vi "JSON String for Simulink Models.vi"() -> ()   [LabVIEW 2018]
uses:
  NistPluggableModules/AcPwr/AcPwrPlugins/ChromaAcLoadClass/TypeDefs/Measurements.ctl
  NistPluggableModules/AcPwr/AcPwrPlugins/ChromaAcLoadClass/TypeDefs/MeasurementType.ctl
  NistPluggableModules/AcPwr/AcPwrShared/clMeasurmentData.ctl
  <vilib>/addons/_JKI.lib/Serialization/JSON/JKI JSON Serialization.lvlib
  NistPluggableModules/AcPwr/AcPwrPlugins/ChromaAcLoadClass/ChromaAcLoad.lvclass
  NistPluggableModules/AcPwr/AcPwrShared/AcPwrShared.lvlib
panel:
  in  "MeasurmentDataCluster":T1={"MeasName"="", "XML Data"="", "WaveformData"=[{"t0"=timestamp(0 s since 1904-01-01), "dt"=1.0, "Y"=[5.0]}, {"t0"=timestamp(0 s since 1904-01-01), "dt"=1.0, "Y"=[10.0]}]}
  in  "Measurements":T2=[{"Handle"="CHROMA0", "Name"="", "Enabled"=TRUE, "Measurement Value"=0.0, "Hold Peak Current Measurement"=FALSE, "btnMeasFetch"=TRUE, "ProtectionStatusString"="", "Measurement Type"=enum."Voltage (Vrms or V)"}, {"Handle"="CHROMA0", "Name"="", "Enabled"=TRUE, "Measurement Value"=0.0, "Hold Peak Current Measurement"=FALSE, "btnMeasFetch"=TRUE, "ProtectionStatusString"="", "Measurement Type"=enum."Current (Arms or A)"}]
  out "JSON String 2":string="{\r\n    \"MeasName\":\"\",\r\n    \"XML Data\":\"\",\r\n    \"WaveformData\":[\r\n                {\r\n            \"t0\":\"1904-01-01T00:00:00.000Z\",\r\n            \"dt\":1.00000000000000,\r\n            \"y\":[\r\n                5.00000000000000\r\n            ]\r\n        },\r\n                {\r\n            \"t0\":\"1904-01-01T00:00:00.000Z\",\r\n            \"dt\":1.00000000000000,\r\n            \"y\":[\r\n                10.0000000000000\r\n            ]\r\n        }\r\n    ]\r\n}"
  out "xml string":string="<Cluster>\r\n<Name>Device(s)Settings</Name>\r\n<NumElts>6</NumElts>\r\n<EW>\r\n<Name>Configuration Mode</Name>\r\n<Choice>Constant Voltage (DC)</Choice>\r\n<Choice>Constant Power (DC)</Choice>\r\n<Choice>Constant Power (AC)</Choice>\r\n<Choice>Constant Current (DC)</Choice>\r\n<Choice>Constant Current (AC)</Choice>\r\n<Choice>Constant Resistance (DC)</Choice>\r\n<Choice>Constant Resistance (AC)</Choice>\r\n<Choice>Rectified Mode (DC)</Choice>\r\n<Choice>Inrush (AC)</Choice>\r\n<Choice>RLC CP (AC)</Choice>\r\n<Choice>RLC (AC)</Choice>\r\n<Val>1</Val>\r\n</EW>\r\n<Array>\r\n<Name>Phases</Name>\r\n<Dimsize>1</Dimsize>\r\n<Cluster>\r\n<Name>Config</Name>\r\n<NumElts>23</NumElts>\r\n<String>\r\n<Name>Handle</Name>\r\n<Val>CHROMA0</Val>\r\n</String>\r\n<String>\r\n<Name>Name</Name>\r\n<Val></Val>\r\n</String>\r\n<I32>\r\n<Name>Phase Select</Name>\r\n<Val>0</Val>\r\n</I32>\r\n<String>\r\n<Name>Instrument Options</Name>\r\n<Val>Simulate=0,RangeCheck=1,QueryInstrStatus=1,Cache=0</Val>\r\n</String>\r\n<Boolean>\r\n<Name>id query (T)</Name>\r\n<Val>1</Val>\r\n</Boolean>\r\n<Boolean>\r\n<Name>reset device (T)</Name>\r\n<Val>1</Val>\r\n</Boolean>\r\n<Boolean>\r\n<Name>Load Short Circuited</Name>\r\n<Val>0</Val>\r\n</Boolean>\r\n<Boolean>\r\n<Name>Line Synchronization</Name>\r\n<Val>0</Val>\r\n</Boolean>\r\n<DBL>\r\n<Name>Load Current (A/Arms)</Name>\r\n<Val>1.00000000000000</Val>\r\n</DBL>\r\n<DBL>\r\n<Name>Load Voltage (V/Vrms)</Name>\r\n<Val>38.00000000000000</Val>\r\n</DBL>\r\n<DBL>\r\n<Name>Load Power (W)</Name>\r\n<Val>5.00000000000000</Val>\r\n</DBL>\r\n<DBL>\r\n<Name>Load Resistance (Ohms)</Name>\r\n<Val>1.50000000000000</Val>\r\n</DBL>\r\n<DBL>\r\n<Name>Load Current Peak Limit (A)</Name>\r\n<Val>45.00000000000000</Val>\r\n</DBL>\r\n<DBL>\r\n<Name>Load Current Limit (A/Arms)</Name>\r\n<Val>10.00000000000000</Val>\r\n</DBL>\r\n<DBL>\r\n<Name>Load Power Limit (W)</Name>\r\n<Val>1250.00000000000000</Val>\r\n</DBL>\r\n<DBL>\r\n<Name>Synch Frequency (Hz)</Name>\r\n<Val>0.00000000000000</Val>\r\n</DBL>\r\n<EW>\r\n<Name>Priority</Name>\r\n<Choice>CF Only</Choice>\r\n<Choice>PF Only</Choice>\r\n<Choice>Both (CF)</Choice>\r\n<Choice>Both (PF)</Choice>\r\n<Val>0</Val>\r\n</EW>\r\n<DBL>\r\n<Name>Crest Factor</Name>\r\n<Val>1.41400000000000</Val>\r\n</DBL>\r\n<DBL>\r\n<Name>Power Factor</Name>\r\n<Val>1.00000000000000</Val>\r\n</DBL>\r\n<Cluster>\r\n<Name>Slew Rate</Name>\r\n<NumElts>2</NumElts>\r\n<I32>\r\n<Name>Rise Slew Rate (A/ms)</Name>\r\n<Val>600</Val>\r\n</I32>\r\n<I32>\r\n<Name>Fall Slew Rate (A/ms)</Name>\r\n<Val>600</Val>\r\n</I32>\r\n</Cluster>\r\n<Cluster>\r\n<Name>LC/RLC Mode</Name>\r\n<NumElts>4</NumElts>\r\n<I32>\r\n<Name>Capacitance (uF)</Name>\r\n<Val>0</Val>\r\n</I32>\r\n<I32>\r\n<Name>Inductance (uH)</Name>\r\n<Val>0</Val>\r\n</I32>\r\n<DBL>\r\n<Name>Series Resistance (Ohm)</Name>\r\n<Val>0.00000000000000</Val>\r\n</DBL>\r\n<DBL>\r\n<Name>Parallel Resistance (Ohm)</Name>\r\n<Val>0.00000000000000</Val>\r\n</DBL>\r\n</Cluster>\r\n<Cluster>\r\n<Name>Timing</Name>\r\n<NumElts>5</NumElts>\r\n<EW>\r\n<Name>TimingOn</Name>\r\n<Choice></Choice>\r\n<Val>0</Val>\r\n</EW>\r\n<U32>\r\n<Name>Hours</Name>\r\n<Val>0</Val>\r\n</U32>\r\n<U32>\r\n<Name>Minutes</Name>\r\n<Val>0</Val>\r\n</U32>\r\n<DBL>\r\n<Name>Seconds</Name>\r\n<Val>0.00000000000000</Val>\r\n</DBL>\r\n<DBL>\r\n<Name>CutoffVoltage</Name>\r\n<Val>0.00000000000000</Val>\r\n</DBL>\r\n</Cluster>\r\n<Boolean>\r\n<Name>Connected</Name>\r\n<Val>0</Val>\r\n</Boolean>\r\n</Cluster>\r\n</Array>\r\n<String>\r\n<Name>MeasName</Name>\r\n<Val>AcPwr.ChromaAcLoad.63804-CH0</Val>\r\n</String>\r\n<String>\r\n<Name>Data Source</Name>\r\n<Val>ICDAS_Simulink_DB</Val>\r\n</String>\r\n<String>\r\n<Name>ICDAS to Model Table Name</Name>\r\n<Val>ICDAS_Simulink_DB</Val>\r\n</String>\r\n<String>\r\n<Name>Model to ICDAS Table Name</Name>\r\n<Val>ICDAS_Simulink_DB</Val>\r\n</String>\r\n</Cluster>\r\n"
  out "JSON String":string="{\r\n    \"Device(s)Settings\":{\r\n        \"Configuration Mode\":1,\r\n        \"Phases\":[\r\n            {\r\n                \"Handle\":\"CHROMA0\",\r\n                \"Name\":\"\",\r\n                \"Phase Select\":0,\r\n                \"Instrument Options\":\"Simulate=0,RangeCheck=1,QueryInstrStatus=1,Cache=0\",\r\n                \"id query (T)\":true,\r\n                \"reset device (T)\":true,\r\n                \"Load Short Circuited\":false,\r\n                \"Line Synchronization\":false,\r\n                \"Load Current (A/Arms)\":1.00000000000000,\r\n                \"Load Voltage (V/Vrms)\":38.0000000000000,\r\n                \"Load Power (W)\":5.00000000000000,\r\n                \"Load Resistance (Ohms)\":1.50000000000000,\r\n                \"Load Current Peak Limit (A)\":45.0000000000000,\r\n                \"Load Current Limit (A/Arms)\":10.0000000000000,\r\n                \"Load Power Limit (W)\":1250.00000000000,\r\n                \"Synch Frequency (Hz)\":0.00000000000000,\r\n                \"Priority\":0,\r\n                \"Crest Factor\":1.41400000000000,\r\n                \"Power Factor\":1.00000000000000,\r\n                \"Slew Rate\":{\r\n                    \"Rise Slew Rate (A/ms)\":600,\r\n                    \"Fall Slew Rate (A/ms)\":600\r\n                },\r\n                \"LC/RLC Mode\":{\r\n                    \"Capacitance (uF)\":0,\r\n                    \"Inductance (uH)\":0,\r\n                    \"Series Resistance (Ohm)\":0.00000000000000,\r\n                    \"Parallel Resistance (Ohm)\":0.00000000000000\r\n                },\r\n                \"Timing\":{\r\n                    \"TimingOn\":0,\r\n                    \"Hours\":0,\r\n                    \"Minutes\":0,\r\n                    \"Seconds\":0.00000000000000,\r\n                    \"CutoffVoltage\":0.00000000000000\r\n                },\r\n                \"Connected\":false\r\n            }\r\n        ],\r\n        \"MeasName\":\"AcPwr.ChromaAcLoad.63804-CH0\",\r\n        \"Data Source\":\"ICDAS_Simulink_DB\",\r\n        \"ICDAS to Model Table Name\":\"ICDAS_Simulink_DB\",\r\n        \"Model to ICDAS Table Name\":\"ICDAS_Simulink_DB\"\r\n    },\r\n    \"Measurements\":[\r\n        {\r\n            \"Handle\":\"CHROMA0\",\r\n            \"Name\":\"\",\r\n            \"Enabled\":true,\r\n            \"Measurement Value\":0.00000000000000,\r\n            \"Hold Peak Current Measurement\":false,\r\n            \"btnMeasFetch\":true,\r\n            \"ProtectionStatusString\":\"\",\r\n            \"Measurement Type\":0\r\n        },\r\n        {\r\n            \"Handle\":\"CHROMA0\",\r\n            \"Name\":\"\",\r\n            \"Enabled\":true,\r\n            \"Measurement Value\":0.00000000000000,\r\n            \"Hold Peak Current Measurement\":false,\r\n            \"btnMeasFetch\":true,\r\n            \"ProtectionStatusString\":\"\",\r\n            \"Measurement Type\":1\r\n        }\r\n    ]\r\n}"
  in  "Device(s)Settings":T4={"Configuration Mode"=enum."Constant Power (DC)", "Phases"=[{"Handle"="CHROMA0", "Name"="", "Phase Select"=0, "Instrument Options"="Simulate=0,RangeCheck=1,QueryInstrStatus=1,Cache=0", "id query (T)"=TRUE, "reset device (T)"=TRUE, "Load Short Circuited"=FALSE, "Line Synchronization"=FALSE, "Load Current (A/Arms)"=1.0, "Load Voltage (V/Vrms)"=38.0, "Load Power (W)"=5.0, "Load Resistance (Ohms)"=1.5, "Load Current Peak Limit (A)"=45.0, "Load Current Limit (A/Arms)"=10.0, "Load Power Limit (W)"=1250.0, "Synch Frequency (Hz)"=0.0, "Priority"=enum."CF Only", "Crest Factor"=1.414, "Power Factor"=1.0, "Slew Rate"={"Rise Slew Rate (A/ms)"=600, "Fall Slew Rate (A/ms)"=600}, "LC/RLC Mode"={"Capacitance (uF)"=0, "Inductance (uH)"=0, "Series Resistance (Ohm)"=0.0, "Parallel Resistance (Ohm)"=0.0}, "Timing"={"TimingOn"=enum."", "Hours"=0, "Minutes"=0, "Seconds"=0.0, "CutoffVoltage"=0.0}, "Connected"=FALSE}], "MeasName"="AcPwr.ChromaAcLoad.63804-CH0", "Data Source"="ICDAS_Simulink_DB", "ICDAS to Model Table Name"="ICDAS_Simulink_DB", "Model to ICDAS Table Name"="ICDAS_Simulink_DB"} {"Phases"."Phase Select" items=["Phase ALL", "Phase A", "Phase B", "Phase C"]}
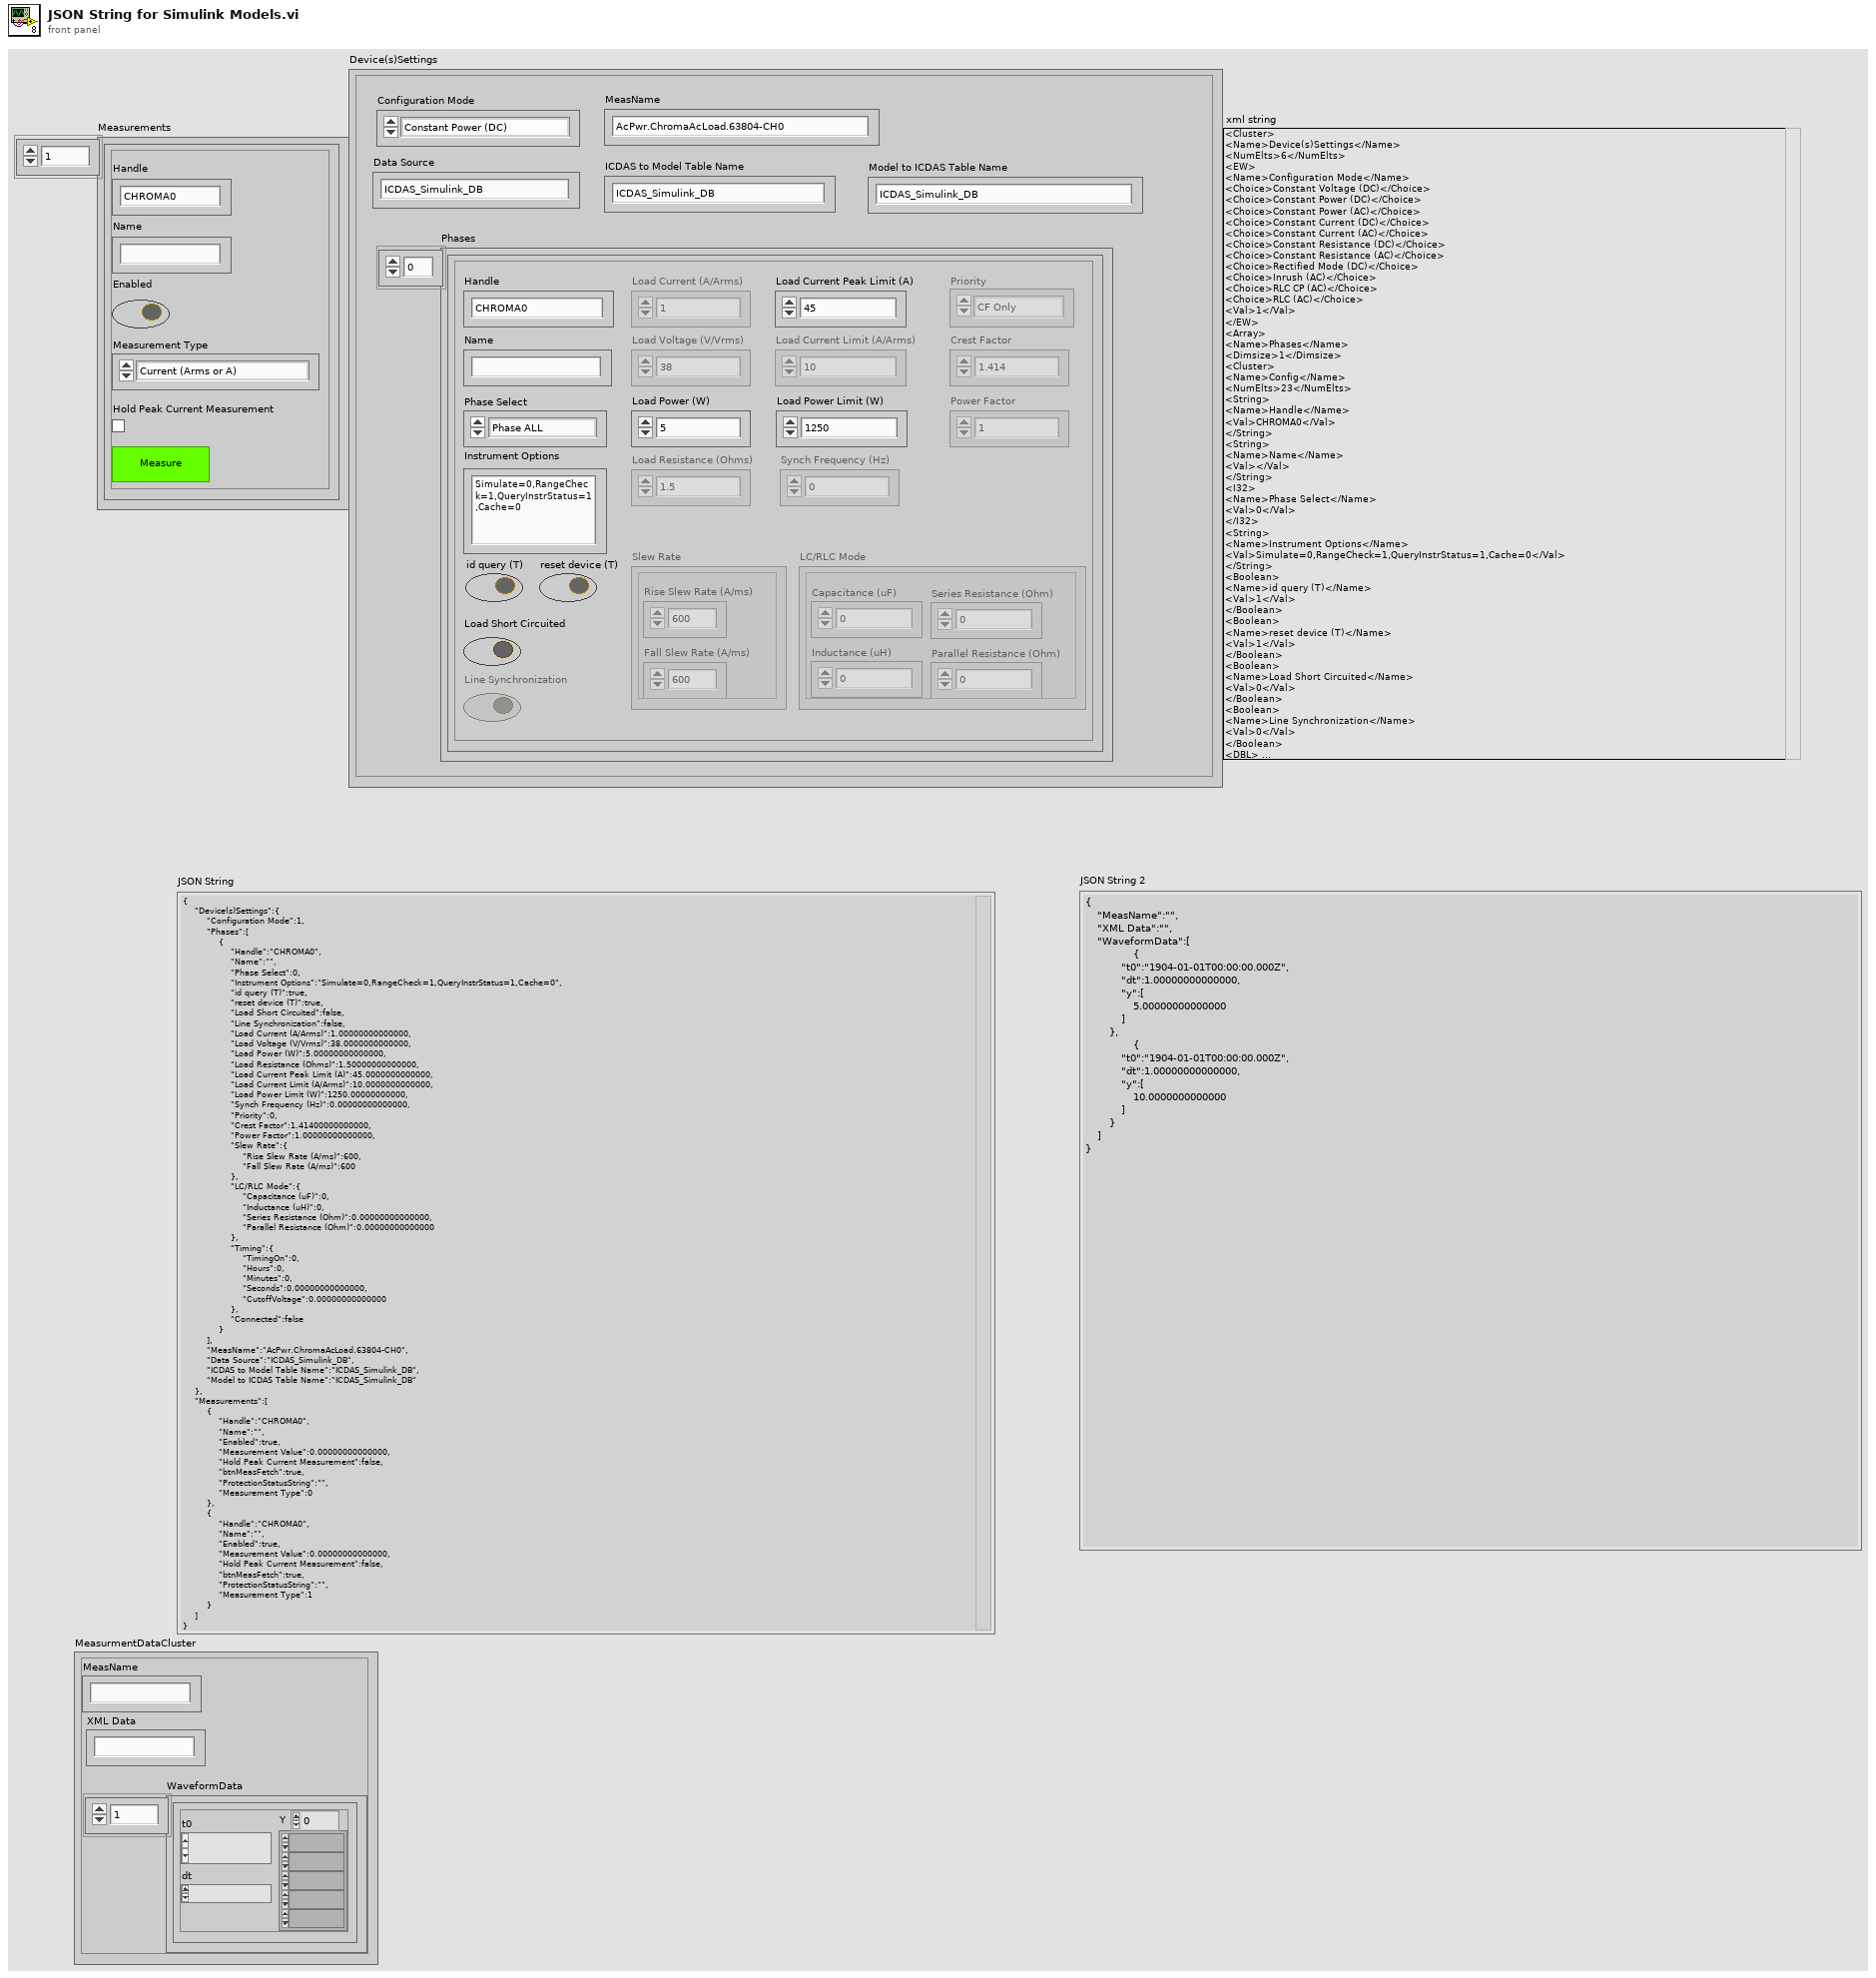
[diagram p1: front panel]
types:
  T1 = typedef "AcPwrShared.lvlib/clMeasurmentData.ctl" = cluster{"MeasName":string, "XML Data":string, "WaveformData":waveform(dbl)[]}
  T2 = typedef "AcPwrPlugins.lvlib/ChromaAcLoad.lvclass/Measurements.ctl" = cluster{"Handle":string, "Name":string, "Enabled":bool, "Measurement Value":dbl, "Hold Peak Current Measurement":bool, "btnMeasFetch":bool, "ProtectionStatusString":string, "Measurement Type":T3}[]
  T3 = typedef "AcPwrPlugins.lvlib/ChromaAcLoad.lvclass/MeasurementType.ctl" = enum16{"Voltage (Vrms or V)", "Current (Arms or A)", "Power (W)", "Peak Voltage (V)", "Peak Current (A)", "Peak Power (W)", "Frequency (Hz)", "Resistance (Ohms)", "Voltage Overshoot (V)", "Positive Peak Current (A)", "Voltage Undershoot (V)", "Negative Peak Current (A)", "Apparent Power (VA)", "Reacitive Power (VAR)", "Voltage THD", "Power Factor", "Current's Crest Factor"}
  T4 = cluster{"Configuration Mode":enum16{"Constant Voltage (DC)", "Constant Power (DC)", "Constant Power (AC)", "Constant Current (DC)", "Constant Current (AC)", "Constant Resistance (DC)", "Constant Resistance (AC)", "Rectified Mode (DC)", "Inrush (AC)", "RLC CP (AC)", "RLC (AC)"}, "Phases":cluster{"Handle":string, "Name":string, "Phase Select":i32, "Instrument Options":string, "id query (T)":bool, "reset device (T)":bool, "Load Short Circuited":bool, "Line Synchronization":bool, "Load Current (A/Arms)":dbl, "Load Voltage (V/Vrms)":dbl, "Load Power (W)":dbl, "Load Resistance (Ohms)":dbl, "Load Current Peak Limit (A)":dbl, "Load Current Limit (A/Arms)":dbl, "Load Power Limit (W)":dbl, "Synch Frequency (Hz)":dbl, "Priority":enum16{"CF Only", "PF Only", "Both (CF)", "Both (PF)"}, "Crest Factor":dbl, "Power Factor":dbl, "Slew Rate":cluster{"Rise Slew Rate (A/ms)":i32, "Fall Slew Rate (A/ms)":i32}, "LC/RLC Mode":cluster{"Capacitance (uF)":i32, "Inductance (uH)":i32, "Series Resistance (Ohm)":dbl, "Parallel Resistance (Ohm)":dbl}, "Timing":cluster{"TimingOn":enum16{""}, "Hours":u32, "Minutes":u32, "Seconds":dbl, "CutoffVoltage":dbl}, "Connected":bool}[], "MeasName":string, "Data Source":string, "ICDAS to Model Table Name":string, "Model to ICDAS Table Name":string}
  T5 = cluster{"Device(s)Settings":cluster{"Configuration Mode":enum16{"Constant Voltage (DC)", "Constant Power (DC)", "Constant Power (AC)", "Constant Current (DC)", "Constant Current (AC)", "Constant Resistance (DC)", "Constant Resistance (AC)", "Rectified Mode (DC)", "Inrush (AC)", "RLC CP (AC)", "RLC (AC)"}, "Phases":cluster{"Handle":string, "Name":string, "Phase Select":i32, "Instrument Options":string, "id query (T)":bool, "reset device (T)":bool, "Load Short Circuited":bool, "Line Synchronization":bool, "Load Current (A/Arms)":dbl, "Load Voltage (V/Vrms)":dbl, "Load Power (W)":dbl, "Load Resistance (Ohms)":dbl, "Load Current Peak Limit (A)":dbl, "Load Current Limit (A/Arms)":dbl, "Load Power Limit (W)":dbl, "Synch Frequency (Hz)":dbl, "Priority":enum16{"CF Only", "PF Only", "Both (CF)", "Both (PF)"}, "Crest Factor":dbl, "Power Factor":dbl, "Slew Rate":cluster{"Rise Slew Rate (A/ms)":i32, "Fall Slew Rate (A/ms)":i32}, "LC/RLC Mode":cluster{"Capacitance (uF)":i32, "Inductance (uH)":i32, "Series Resistance (Ohm)":dbl, "Parallel Resistance (Ohm)":dbl}, "Timing":cluster{"TimingOn":enum16{""}, "Hours":u32, "Minutes":u32, "Seconds":dbl, "CutoffVoltage":dbl}, "Connected":bool}[], "MeasName":string, "Data Source":string, "ICDAS to Model Table Name":string, "Model to ICDAS Table Name":string}, "Measurements":T2}
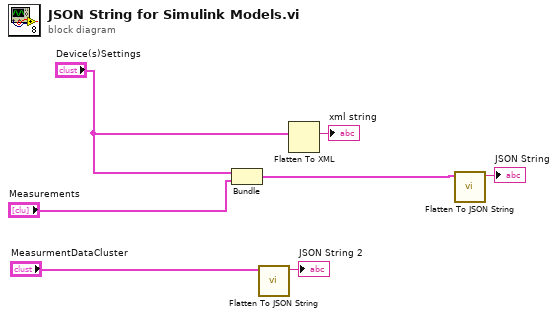
[diagram p0: block diagram]
diagram:
  n1 = Bundle("Device(s)Settings"="Device(s)Settings", "Measurements"="Measurements") -> (w1:T5)  [unwired: 1 in]
  n2 = call <vilib>:"Flatten To JSON String.vi"("Variant"="MeasurmentDataCluster") -> ("JSON String"=→"JSON String 2":string)  [unwired: 9 in, 1 out]
  n3 = Flatten To XML(anything="Device(s)Settings") -> (xml string=→"xml string":string)
  n4 = call <vilib>:"Flatten To JSON String.vi"("Variant"=w1) -> ("JSON String"=→"JSON String":string)  [unwired: 9 in, 1 out]
